vi "Run All.vi"(8 "Error In":errorcluster) -> (0 "Error Out":errorcluster)   [LabVIEW 2017, in "Tests.lvlib" / "Reader.lvlib"]
uses:
  Reader.lvlib
  <vilib>/addons/_JKI Toolkits/Caraya/classes/Test/Test.lvclass
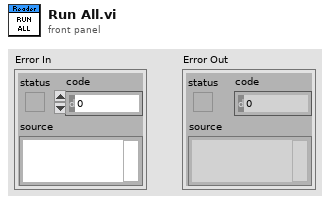
[diagram p1: front panel]
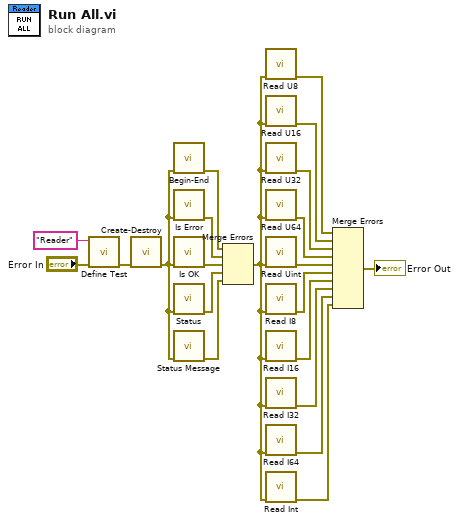
[diagram p0: block diagram]
diagram:
  n1 = call <vilib>:"Define Test.vi"("error in (no error)"="Error In", "Label (VI Title)"="Reader") -> ("error out"=w18:errorcluster)  [unwired: 9 in]
  n2 = call "Create-Destroy.vi"("Error In"=w18) -> ("Error Out"=w14:errorcluster)  [unwired: 10 in]
  n3 = call "Begin-End.vi"("Error In"=w14) -> ("Error Out"=w19:errorcluster)  [unwired: 10 in]
  n4 = call "Is Error.vi"("Error In"=w14) -> ("Error Out"=w17:errorcluster)  [unwired: 10 in]
  n5 = call "Is OK.vi"("Error In"=w14) -> ("Error Out"=w16:errorcluster)  [unwired: 10 in]
  n6 = call "Status.vi"("Error In"=w14) -> ("Error Out"=w15:errorcluster)  [unwired: 10 in]
  n7 = call "Status Message.vi"("Error In"=w14) -> ("Error Out"=w13:errorcluster)  [unwired: 10 in]
  n8 = Merge Errors(w19, w17, w16, w15, w13) -> (w2:errorcluster)
  n9 = call "Read U8.vi"("Error In"=w2) -> ("Error Out"=w12:errorcluster)  [unwired: 10 in]
  n10 = call "Read U16.vi"("Error In"=w2) -> ("Error Out"=w10:errorcluster)  [unwired: 10 in]
  n11 = call "Read U32.vi"("Error In"=w2) -> ("Error Out"=w9:errorcluster)  [unwired: 10 in]
  n12 = call "Read U64.vi"("Error In"=w2) -> ("Error Out"=w8:errorcluster)  [unwired: 10 in]
  n13 = call "Read Uint.vi"("Error In"=w2) -> ("Error Out"=w7:errorcluster)  [unwired: 10 in]
  n14 = call "Read I8.vi"("Error In"=w2) -> ("Error Out"=w6:errorcluster)  [unwired: 10 in]
  n15 = call "Read I16.vi"("Error In"=w2) -> ("Error Out"=w5:errorcluster)  [unwired: 10 in]
  n16 = call "Read I32.vi"("Error In"=w2) -> ("Error Out"=w4:errorcluster)  [unwired: 10 in]
  n17 = call "Read I64.vi"("Error In"=w2) -> ("Error Out"=w3:errorcluster)  [unwired: 10 in]
  n18 = call "Read Int.vi"("Error In"=w2) -> ("Error Out"=w1:errorcluster)  [unwired: 10 in]
  n19 = Merge Errors(w12, w10, w9, w8, w7, w6, w5, w4, w3, w1) -> (→"Error Out":errorcluster)
